vi "Merge PGM Map.vi"(8 "error in (no error)":errorcluster, 11 "Map Model in":refnum<class "Map Model.lvclass">) -> (0 "error out":errorcluster, 1 "Map Rectangle":T1, 2 "Map":picture, 3 "Map Model out":refnum<class "Map Model.lvclass">)   [LabVIEW 2020, in "Map Model.lvlib" / "Map Model.lvclass"]
uses:
  Map Model.lvclass
  Map Model.lvclass/Map Model.ctl
panel:
  # "NOTICE -- YOU MUST LEAVE THIS NOTICE IN PLACE.\n\nCopyright (c) 2017, LIANG LIU Shawn.Liu.cn@gmail.com\nAll rights reserved.\n\nRedistribution and use in source and binary forms, with or without modification, are permitted provided that the following conditions are met:\n-Redistributions of source code must retain the above copyright notice, this list of conditions and the following disclaimer.\n-Redistributions in binary form must reproduce the above copyright notice, this list of conditions and the following disclaimer in the documentation and/or other materials provided with the distribution.\n-Neither the name of the eLp nor the names of its contributors may be used to endorse or promote products derived from this software without specific prior written permission.\n\nTHIS SOFTWARE IS PROVIDED BY THE COPYRIGHT HOLDERS AND CONTRIBUTORS \"AS IS\" AND ANY EXPRESS OR IMPLIED WARRANTIES, INCLUDING, BUT NOT LIMITED TO, THE IMPLIED WARRANTIES OF MERCHANTABILITY AND FITNESS FOR A PARTICULAR PURPOSE ARE DISCLAIMED. IN NO EVENT SHALL THE COPYRIGHT HOLDER OR CONTRIBUTORS BE LIABLE FOR ANY DIRECT, INDIRECT, INCIDENTAL, SPECIAL, EXEMPLARY, OR CONSEQUENTIAL DAMAGES (INCLUDING, BUT NOT LIMITED TO, PROCUREMENT OF SUBSTITUTE GOODS OR SERVICES; LOSS OF USE, DATA, OR PROFITS; OR BUSINESS INTERRUPTION) HOWEVER CAUSED AND ON ANY THEORY OF LIABILITY, WHETHER IN CONTRACT, STRICT LIABILITY, OR TORT (INCLUDING NEGLIGENCE OR OTHERWISE) ARISING IN ANY WAY OUT OF THE USE OF THIS SOFTWARE, EVEN IF ADVISED OF THE POSSIBILITY OF SUCH DAMAGE."
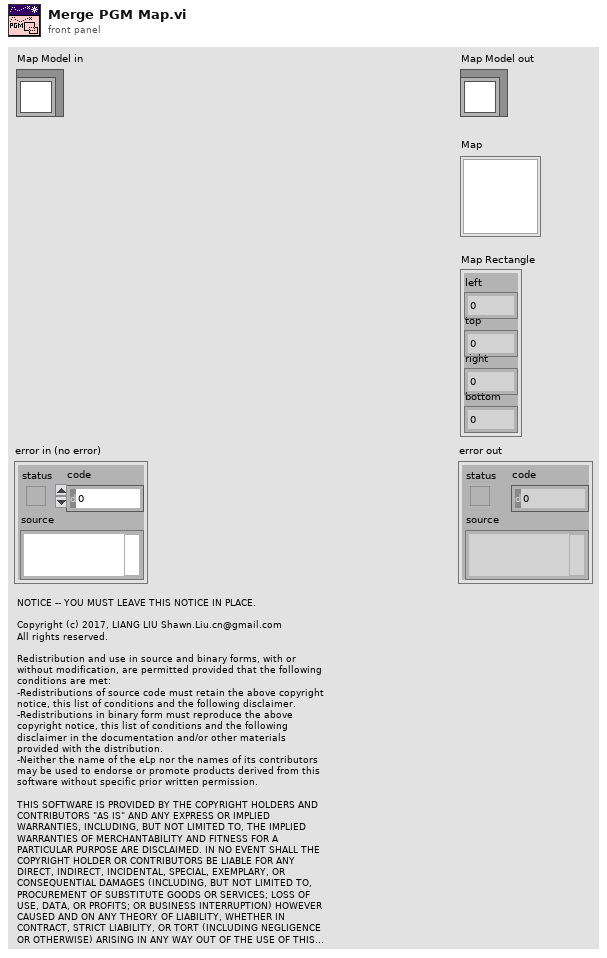
[diagram p1: front panel]
types:
  T1 = cluster{"left":i16, "top":i16, "right":i16, "bottom":i16}
  T2 = typedef "imagedata.ctl" = cluster{"image type":i32, "image depth":i32, "image":u8[], "mask":u8[], "colors":u32[], "Rectangle":cluster{"left":i16, "top":i16, "right":i16, "bottom":i16}}
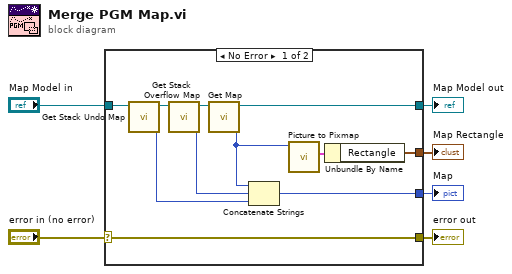
[diagram p0: block diagram]
diagram:
  n1 = case shown="No Error" "error in (no error)" {
    selector: "error in (no error)" -> [w14 w19]
    tunnel: [w17 _] -> w6
    tunnel: [w16 w18] -> w5
    tunnel: "Map Model in" -> [w15 w18]
    tunnel: [w7 _] -> w2
    tunnel: [w14 w19] -> w1
    frame No Error {
      n2 = call "Get Stack Undo Map.vi"("Map Model in"=w15) -> ("Stack Undo Map"=w12:picture, "Map Model out"=w11:refnum<class "Map Model.lvclass">)  [unwired: 9 in]
      n3 = call "Get Stack Overflow Map.vi"("Map Model in"=w11) -> ("Stack Overflow Map"=w13:picture, "Map Model out"=w10:refnum<class "Map Model.lvclass">)  [unwired: 9 in]
      n4 = call "Get Map.vi"("Map Model in"=w10) -> ("Map"=w8:picture, "Map Model out"=w16:refnum<class "Map Model.lvclass">)  [unwired: 9 in]
      n5 = Concatenate Strings(w8, w13, w12) -> (w17:picture)
      n6 = call <vilib>:"Picture to Pixmap.vi"("picture"=w8) -> ("image data"=w9:T2)  [unwired: 9 in, 1 out]
      n7 = Unbundle By Name(w9) -> ("Rectangle"=w7:T1)
    }
    frame Error {
    }
  }
  "error out" <- w1
  "Map Model out" <- w5
  "Map" <- w6
  "Map Rectangle" <- w2
